vi "Image_aquire(subVI).vi"(8 "error in":errorcluster, 10 "Image Type":T1 items=["Grayscale (U8)", "Grayscale (I16)", "Grayscale (SGL)", "Complex (CSG)", "RGB (U32)", "HSL (U32)", "RGB (U64)", "Grayscale (U16)"], 11 "Session In":T2="cam0") -> (0 "error out":errorcluster, 2 "RGB image":T3(plugin-control), 3 "Grey scale image":T3(plugin-control))   [LabVIEW 2020]
doc: "Acquisice l'immagine di una telecamera a colori e la restituisce in bianco e nero."
uses:
  <vilib>/userdefined/High Color/IMAQdx.ctl
  <vilib>/vision/driver/NI_Vision_Acquisition_Software.lvlib
panel:
  in  "stop":bool
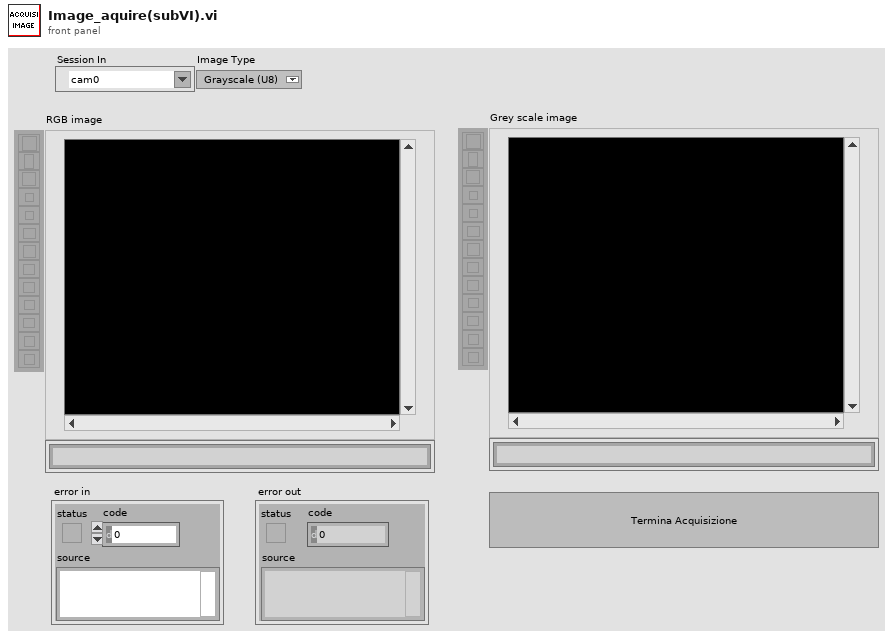
[diagram p1: front panel]
types:
  T1 = typedef "Image Type" = u32
  T2 = typedef "IMAQdx.ctl" = refnum<k21>
  T3 = typedef "IMAQ Image.ctl" = refnum<image>
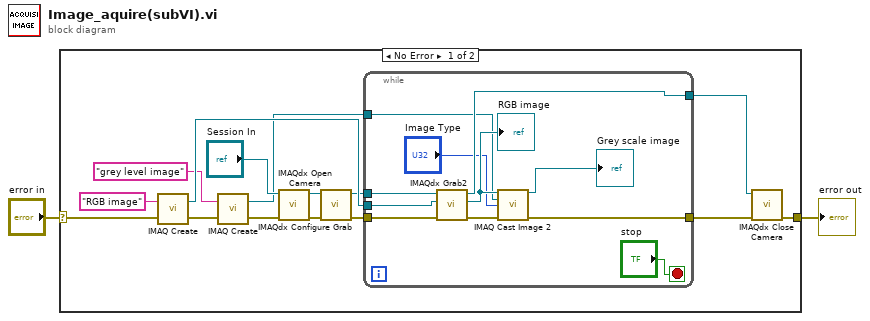
[diagram p0: block diagram]
diagram:
  n1 = case shown="No Error" "error in" {
    selector: "error in" -> [w4 w29]
    tunnel: [w9 w29] -> w2
    frame No Error {
      n2 = call "IMAQ Create"("Image Name"="RGB image", "error in (no error)"=w4) -> ("New Image"=w13:T3, "error out"=w8:errorcluster)  [unwired: 3 in]
      n3 = call "IMAQ Create"("Image Name"="grey level image", "error in (no error)"=w8) -> ("New Image"=w5:T3, "error out"=w7:errorcluster)  [unwired: 3 in]
      n4 = call <vilib>:"IMAQdx Open Camera.vi"("error in"=w7, "Session In"="Session In") -> ("error out"=w15:errorcluster, "Session Out"=w16:T2)  [unwired: 8 in]
      n5 = call <vilib>:"IMAQdx Configure Grab.vi"("error in"=w15, "Session In"=w16) -> ("error out"=w10:errorcluster, "Session Out"=w12:T2)  [unwired: 8 in]
      n6 = while {
        tunnel: w13 -> [w28]
        tunnel: w12 -> [w27]
        tunnel: [w25] -> w11
        tunnel: w10 -> [w24]
        tunnel: [w21] -> w3
        tunnel: w5 -> [w19]
        stop <- "stop" stop-if-true
        n7 = call <vilib>:"IMAQdx Grab2.vi"("error in"=w24, "Image In"=w28, "Session In"=w27) -> ("error out"=w22:errorcluster, "Image Out"=w23:T3, "Session Out"=w25:T2)  [unwired: 5 in, 1 out]
        "RGB image" <- w23
        n8 = call "IMAQ Cast Image 2"("Image Src"=w23, "Image Dst"=w19, "Image Type"="Image Type", "error in (no error)"=w22) -> ("Image Dst Out"=→"Grey scale image":T3, "error out"=w21:errorcluster)  [unwired: 10 in]
      }
      n9 = call <vilib>:"IMAQdx Close Camera.vi"("error in"=w3, "Session In"=w11) -> ("error out"=w9:errorcluster)  [unwired: 9 in]
    }
    frame Error {
    }
  }
  "error out" <- w2
